vi "C(T) data packer.vi"(0 "Path in":path=path "C:/Documents and Settings/pk/My Documents/P350/P350 F01/P350 F01 Instructor/Projects w sol/P5/P350 C(T) experimental data file 11 06 01 c.txt", 1 "launch viewer":bool=TRUE, 5 "Temp Array In":dbl[](array[numeric])=[26.0, 30.0, 34.0, 38.0, 42.0, 46.0, 50.0] format="%.2f", 7 "Timing Control Parameters In":T1={"N cycles for averaging"=100, "N points per measurement"=1000, "Measurment time interval"=2e-05} {"Measurment time interval" format="%.2e"}, 9 "Data In":waveform(dbl)[](array[waveform])=[{"t0"=timestamp(3087922235.213 s since 1904-01-01), "dt"=1.9999999494757503e-05, "Y"=array[1000 elements]}, {"t0"=timestamp(3087922405.147 s since 1904-01-01), "dt"=1.9999999494757503e-05, "Y"=array[1000 elements]}, {"t0"=timestamp(3087922549.515 s since 1904-01-01), "dt"=1.9999999494757503e-05, "Y"=array[1000 elements]}, {"t0"=timestamp(3087922690.9379997 s since 1904-01-01), "dt"=1.9999999494757503e-05, "Y"=array[1000 elements]}, {"t0"=timestamp(3087922829.417 s since 1904-01-01), "dt"=1.9999999494757503e-05, "Y"=array[1000 elements]}, {"t0"=timestamp(3087922967.796 s since 1904-01-01), "dt"=1.9999999494757503e-05, "Y"=array[1000 elements]}, {"t0"=timestamp(3087923101.799 s since 1904-01-01), "dt"=1.9999999494757503e-05, "Y"=array[1000 elements]}], 11 "error in":errorcluster) -> (4 "Path out":path=path "C:/Documents and Settings/pk/My Documents/P350/P350 F01/P350 F01 Instructor/Projects w sol/P5/P350 C(T) experimental data file 11 06 01 c.txt", 8 "data spreadsheet":dbl[][](array[numeric]) format="%.2e", 13 "no save out":bool, 15 "error out":errorcluster)   [LabVIEW 2014]
doc: "This vi manages the data processing and data viewing process after acquisition.\n\nPaul K Dixon\nPhysics 350\nCSUSB Physics"
uses:
  globals/C(T) global variables.vi
panel:
  in  "Resistance (Ohms)":dbl=100000.0 format="%.4e"
  out "N temps":i32=7
  # "C(T) Data Packer"
  # "t params"
  # "N temps"
  # "temps"
  # "est caps"
  # "RC decays - - - - - -"
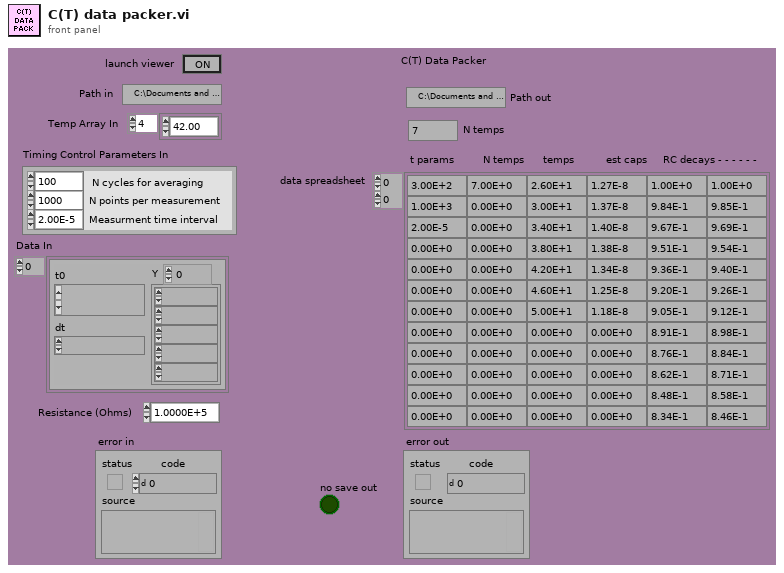
[diagram p1: front panel]
types:
  T1 = cluster{"N cycles for averaging":i32, "N points per measurement":i32, "Measurment time interval":dbl}
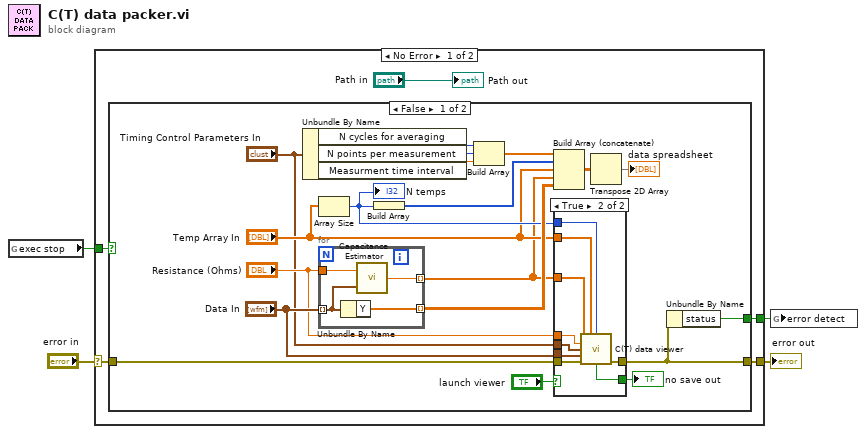
[diagram p0: block diagram]
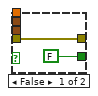
[diagram p2: hidden frame]
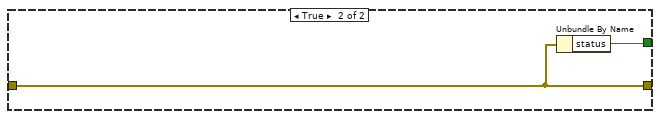
[diagram p3: hidden frame]
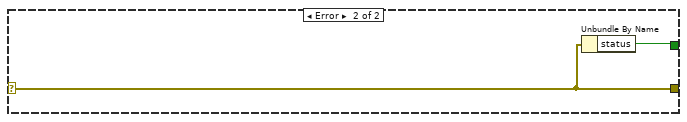
[diagram p4: hidden frame]
diagram:
  n1 = global read "C(T) global variables.vi" "exec stop"() -> (w2:bool)
  n2 = case shown="No Error" "error in" {
    selector: "error in" -> [w9 w46]
    tunnel: [w8 w46] -> w3
    tunnel: w2 -> [w6 _]
    tunnel: [w5 w47] -> w1
    frame No Error {
      n3 = case shown="False" w6 {
        tunnel: w9 -> [w14 w44]
        tunnel: [w11 w44] -> w8
        tunnel: [w10 w45] -> w5
        frame False {
          n4 = Unbundle By Name("Timing Control Parameters In") -> ("N cycles for averaging"=w26:i32, "N points per measurement"=w27:i32, "Measurment time interval"=w28:dbl)
          n5 = Array Size(array="Temp Array In") -> (size(s)=w19:i32)
          "N temps" <- w19
          n6 = for {
            tunnel: "Data In" -> [w42] mode=indexing
            tunnel: [w43] -> w21 mode=indexing
            tunnel: "Resistance (Ohms)" -> [w41]
            tunnel: [w40] -> w17 mode=indexing
            n7 = Unbundle By Name(w42) -> ("Y"=w43:dbl[])
            n8 = call "Capacitance Estimator.vi"("normalized waveform"=w42, "Resistance (Ohms)"=w41) -> ("Estimated Capacitance (F)"=w40:dbl)
          }
          n9 = Build Array(w19) -> (w22:i32[])
          n10 = Build Array(w26, w27, w28) -> (w23:dbl[])
          n11 = Build Array (concatenate)(w23, w22, "Temp Array In", w17, w21) -> (w25:dbl[][])
          n12 = case shown="True" "launch viewer" {
            tunnel: "Data In" -> [_ w39]
            tunnel: w19 -> [_ w38]
            tunnel: "Temp Array In" -> [_ w37]
            tunnel: w17 -> [_ w36]
            tunnel: "Resistance (Ohms)" -> [_ w35]
            tunnel: "Timing Control Parameters In" -> [_ w34]
            tunnel: w14 -> [w30 w33]
            tunnel: [w30 w32] -> w11
            tunnel: [FALSE ("no save out") w31] -> w12
            frame False {
            }
            frame True {
              n13 = call "C(T) data viewer.vi"("Cap Estimates"=w36, "Temps"=w37, "N Temps"=w38, "Resistance (Ohms)"=w35, "Timing Control Parameters"=w34, "waveforms"=w39, "error in"=w33) -> ("no save out"=w31:bool, "error out"=w32:errorcluster)  [unwired: 7 out]
            }
          }
          "no save out" <- w12
          n14 = Transpose 2D Array(2D array=w25) -> (transposed array=→"data spreadsheet":dbl[][])
          n15 = Unbundle By Name(w11) -> ("status"=w10:bool)
        }
        frame True {
          n16 = Unbundle By Name(w44) -> ("status"=w45:bool)
        }
      }
      "Path out" <- "Path in"
    }
    frame Error {
      n17 = Unbundle By Name(w46) -> ("status"=w47:bool)
    }
  }
  "error out" <- w3
  n18 = global write "C(T) global variables.vi" "error detect"(w1) -> ()
